vi "DataGrabber1.vi"(0 "# Images In":u16=208 min=1 max=10000, 1 "Camera Handle":u32=16842752, 2 "error in (no error)":errorcluster) -> (3 "# Images In":u16=208 min=1 max=10000, 4 "Camera Handle":u32, 5 "Data":dbl[][](array[numeric]), 6 "error out":errorcluster)   [LabVIEW 2014]
panel:
  in  "Exposure":dbl=1e-05 min=0.0 step=1e-06 format="%.7f"
  out "Data Graph":sgl[][](graph)
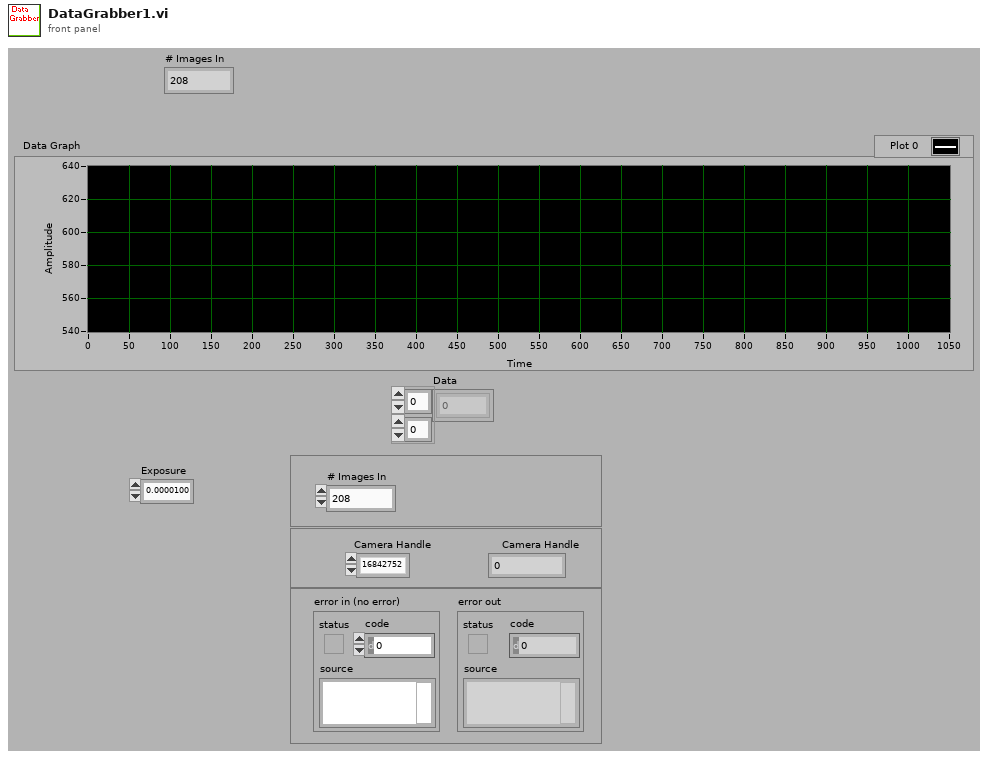
[diagram p1: front panel]
types:
  T1 = cluster{"acquire focus mode":u32, "Exposure":dbl, "# Images In":u16, "Software accumulation":u32}
  T2 = cluster{"Camera Handle":u32, "Pulser Handle":u32, "File Handle":u32, "Display Handle":u32, "Image Handle":u32}
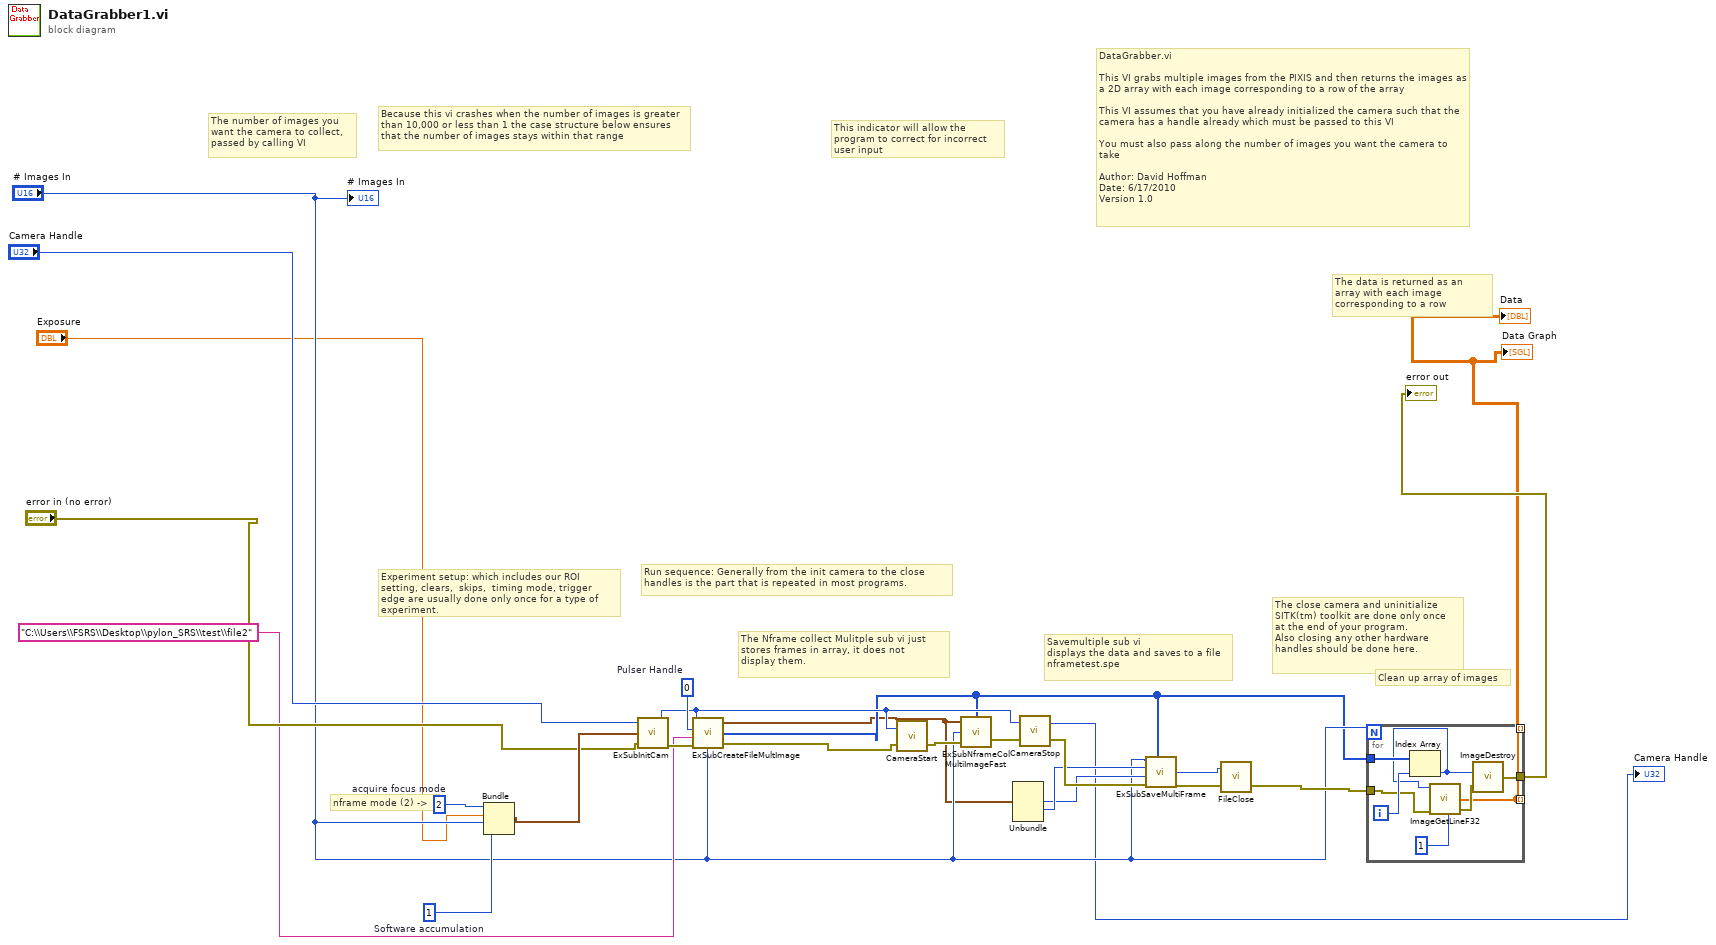
[diagram p0: block diagram]
diagram:
  w22 = u32 0  # Pulser Handle
  w24 = u32 2  # acquire focus mode
  w23 = u32 1  # Software accumulation
  # "Clean up array of images"
  # "Savemultiple sub vi\ndisplays the data and saves to a file\nnframetest.spe"
  # "The Nframe collect Mulitple sub vi just \nstores frames in array, it does not \ndisplay them."
  # "The close camera and uninitialize\nSITK(tm) toolkit are done only once\nat the end of your program.\nAlso closing any other hardware \nhandles should be done here."
  # "Run sequence: Generally from the init camera to the close \nhandles is the part that is repeated in most programs."
  # "Experiment setup: which includes our ROI setting, clears,  skips,  timing mode, trigger edge are usually done only once for a type of experiment."
  # "nframe mode (2) ->"
  # "This indicator will allow the program to correct for incorrect user input"
  # "Because this vi crashes when the number of images is greater than 10,000 or less than 1 the case structure below ensures that the number of images stays within that range"
  # "The data is returned as an array with each image corresponding to a row"
  # "DataGrabber.vi\n\nThis VI grabs multiple images from the PIXIS and then returns the images as a 2D array with each image corresponding to a row of the array\n\nThis VI assumes that you have already initialized the camera such that the camera has a handle already which must be passed to this VI\n\nYou must also pass along the number of images you want the camera to take\n\nAuthor: David Hoffman\nDate: 6/17/2010\nVersion 1.0"
  # "The number of images you want the camera to collect, passed by calling VI"
  n1 = Bundle("acquire focus mode"=w24, "Exposure"="Exposure", "# Images In"="# Images In", "Software accumulation"=w23) -> (w13:T1)  [unwired: 1 in]
  n2 = call "ExSubInitCam.vi"("error in (no error)"="error in (no error)", "Camera Information"=w13, "Camera Handle"="Camera Handle") -> ("error out"=w25:errorcluster, "Camera Handle"=w19:u32)
  n3 = call "ExSubCreateFileMultImage.vi"("Camera Handle"=w19, "Pulser Handle"=w22, "File and Display Name"="C:\\Users\\FSRS\\Desktop\\pylon_SRS\\test\\file2", "error in (no error)"=w25, "Number of Images"="# Images In") -> ("Handles Out"=w1:T2, "Array"=w2:u32[], "error out"=w3:errorcluster)
  n4 = call <userlib>:"CameraStart.vi"("error in"=w3, "Camera Handle"=w19) -> ("error out"=w21:errorcluster)  [unwired: 1 out]
  n5 = call "ExSubNframeColMultiImageFast.vi"("image handles"=w2, "error in (no error)"=w21, "Number of Images"="# Images In", "Handle Cluster"=w1) -> ("error out"=w20:errorcluster)  [unwired: 1 out]
  n6 = Unbundle(w1) -> ("File Handle"=w16:u32, "Display Handle"=w17:u32)  [unwired: 3 out]
  n7 = call <userlib>:"CameraStop.vi"("error in"=w20, "Camera Handle"=w19) -> ("error out"=w18:errorcluster, "Camera Handle"=→"Camera Handle":u32)
  n8 = call "ExSubSaveMultiFrame.vi"("Number of Images"="# Images In", "Display Handle"=w17, "file handle"=w16, "error in (no error)"=w18, "Data handles"=w2) -> ("file Handle"=w5:u32, "error out"=w15:errorcluster)  [unwired: 1 out]
  n9 = call <userlib>:"FileClose.vi"("error in"=w15, "File Handle"=w5) -> ("error out"=w14:errorcluster)
  n10 = for {
    N: "# Images In" -> [_]
    tunnel: w14 -> [w29]
    tunnel: [w33] -> w7
    tunnel: w2 -> [w31]
    tunnel: [w27] -> _ mode=indexing
    tunnel: [w27] -> w6 mode=indexing
    i -> [w32]
    w30 = u32 1
    n11 = Index Array(array=w31, index=w32) -> (element=w26:u32)
    n12 = call <userlib>:"ImageGetLineF32.vi"("error in"=w29, "Z Position"=w30, "Y Position"=w30, "Data Handle"=w26) -> ("error out"=w28:errorcluster, "Array F32"=w27:sgl[])  [unwired: 1 out]
    n13 = call <userlib>:"ImageDestroy.vi"("error in"=w28, "Data handle"=w26) -> ("error out"=w33:errorcluster)
  }
  "error out" <- w7
  "Data" <- w6
  "Data Graph" <- w6
  "# Images In" <- "# Images In"
